vi "Move both motors.vi"(6 "Avance (°)":dbl=1.0 caption="Avance" format="%#_g°", 7 "Current position":cluster{"M1 pos":dbl, "M2 pos ":dbl}, 8 "error in (no error)":errorcluster, 9 "M1 half/full speed (half = 1)":bool, 10 "Motor params":T4, 11 "DAQ Module ID":i32) -> (0 "error out":errorcluster, 3 "Motor control out":T1, 5 "Acq args":T2)   [LabVIEW 2020]
uses:
  controls/Motor direction ---typedef.ctl
  Controls/Motor controls---typedef.ctl
  controls/Continuous acquisition ---argument.ctl
  controls/Motor FGV states ---typedef.ctl
  controls/Motor params ---typedef.ctl
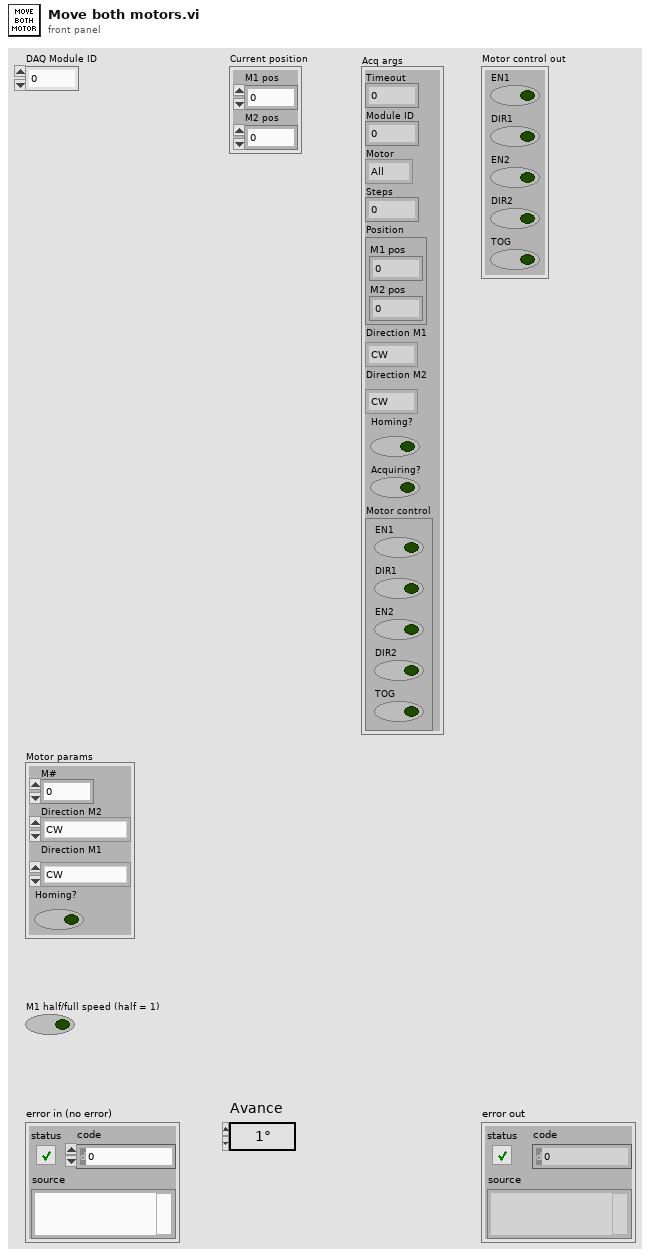
[diagram p1: front panel]
types:
  T1 = typedef "Motor controls---typedef.ctl" = cluster{"EN1":bool, "DIR1":bool, "EN2":bool, "DIR2":bool, "TOG":bool}
  T2 = typedef "Continuous acquisition ---argument.ctl" = cluster{"Timeout":i32, "Module ID":i32, "Motor":enum16{"All", "M1", "M2"}, "Steps":i32, "Position":cluster{"M1 pos":dbl, "M2 pos ":dbl}, "Direction M1":T3, "Direction M2":T3, "Homing?":bool, "Acquiring?":bool, "Motor control":T1}
  T3 = typedef "Motor direction ---typedef.ctl" = enum16{"CW", "CCW", "IDLE"}
  T4 = typedef "Motor params ---typedef.ctl" = cluster{"M#":i32, "Direction M2":T3, "Direction M1":T3, "Homing?":bool}
  T5 = typedef "Motor FGV states ---typedef.ctl" = enum16{"Set", "Reset", "Get"}
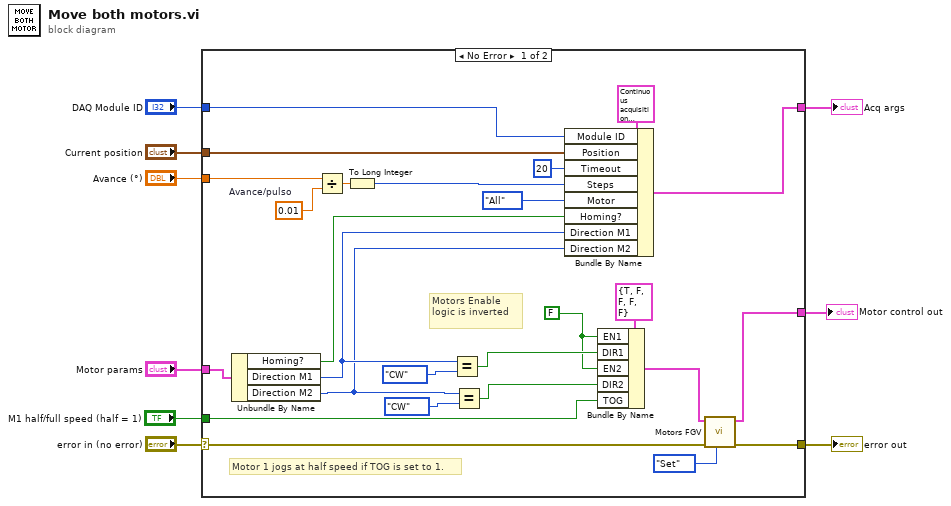
[diagram p0: block diagram]
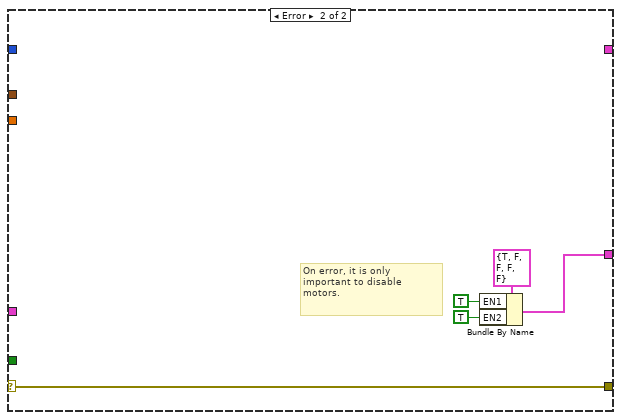
[diagram p2: hidden frame]
diagram:
  n1 = case shown="No Error" "error in (no error)" {
    selector: "error in (no error)" -> [w23 w40]
    tunnel: [w22 w40] -> w9
    tunnel: "DAQ Module ID" -> [w26 _]
    tunnel: "Motor params" -> [w34 _]
    tunnel: "Avance (°)" -> [w33 _]
    tunnel: [w27 _] -> w4
    tunnel: "M1 half/full speed (half = 1)" -> [w24 _]
    tunnel: "Current position" -> [w18 _]
    tunnel: [w14 w36] -> w1
    frame No Error {
      w13 = FALSE ("EN1")
      w32 = 0.01  # Avance/pulso
      # "Motor 1 jogs at half speed if TOG is set to 1."
      # "Motors Enable logic is inverted"
      n2 = Unbundle By Name(w34) -> ("Homing?"=w19:bool, "Direction M1"=w17:T3, "Direction M2"=w10:T3)
      n3 = Divide(x=w33, y=w32) -> (x/y=w31:dbl)
      n4 = To Long Integer(number=w31) -> (32bit integer=w30:i32)
      n5 = Equal?(x=w17, y=Motor_direction_---typedef."CW") -> (x = y?=w15:bool)
      n6 = Equal?(x=w10, y=Motor_direction_---typedef."CW") -> (x = y?=w11:bool)
      n7 = Bundle By Name(cluster=T2 {"Timeout"=0, "Module ID"=0, "Motor"=enum."All", "Steps"=0, "Position"={"M1 pos"=0.0, "M2 pos "=0.0}, "Direction M1"=enum."CW", "Direction M2"=enum."CW", "Homing?"=FALSE, "Acquiring?"=FALSE, "Motor control"={"EN1"=FALSE, "DIR1"=FALSE, "EN2"=FALSE, "DIR2"=FALSE, "TOG"=FALSE}} ("event data"), "Module ID"=w26, "Position"=w18, "Timeout"=20, "Steps"=w30, "Motor"=enum16{"All", "M1", "M2"}."All", "Homing?"=w19, "Direction M1"=w17, "Direction M2"=w10) -> (w27:T2)
      n8 = Bundle By Name(cluster=T1 {"EN1"=TRUE, "DIR1"=FALSE, "EN2"=FALSE, "DIR2"=FALSE, "TOG"=FALSE} ("Motor control"), "EN1"=w13, "DIR1"=w15, "EN2"=w13, "DIR2"=w11, "TOG"=w24) -> (w21:T1)
      n9 = call "Motors FGV.vi"("Action"=Motor_FGV_states_---typedef."Set", "error in (no error)"=w23, "Motor control in"=w21) -> ("error out"=w22:errorcluster, "Motor control out"=w14:T1)  [unwired: 7 in]
    }
    frame Error {
      # "On error, it is only important to disable motors."
      n10 = Bundle By Name(cluster=T1 {"EN1"=TRUE, "DIR1"=FALSE, "EN2"=FALSE, "DIR2"=FALSE, "TOG"=FALSE} ("Motor control"), "EN1"=TRUE, "EN2"=TRUE) -> (w36:T1)
    }
  }
  "error out" <- w9
  "Acq args" <- w4
  "Motor control out" <- w1
